vi "Enable function.vi"(8 "error in (no error)":errorcluster, 10 "Enable function channel?":bool, 11 "VISA resource name":refnum<visa-resource-name>) -> (0 "error out":errorcluster, 3 "VISA resource name out":refnum<visa-resource-name>)   [LabVIEW 2017, in "Sefram DAS220.lvlib"]
doc: "Enable the ability to calculate function between channels (FA1-FJ4 group)."
uses:
  <instrlib>/Sefram DAS220/Sefram DAS220.lvlib
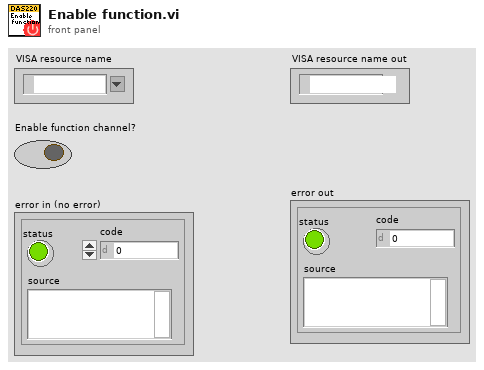
[diagram p1: front panel]
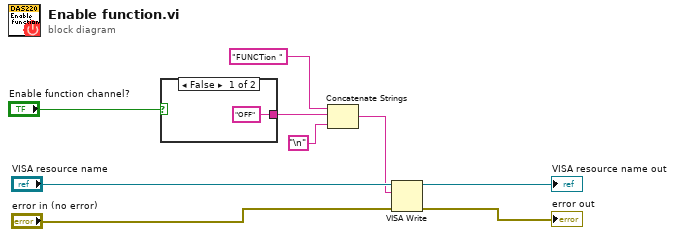
[diagram p0: block diagram]
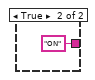
[diagram p2: hidden frame]
diagram:
  n1 = case shown="False" "Enable function channel?" {
    tunnel: ["OFF" "ON"] -> w5
    frame False {
    }
    frame True {
    }
  }
  n2 = Concatenate Strings("FUNCTion " ("string"), w5, "\n") -> (w3:string)
  n3 = VISA Write(VISA resource name="VISA resource name", write buffer=w3, error in (no error)="error in (no error)") -> (VISA resource name out=→"VISA resource name out":refnum<visa-resource-name>, error out=→"error out":errorcluster)  [unwired: 1 out]
